vi "Lissage de signal_base_GJE.vi"() -> ()   [LabVIEW 2018]
panel:
  in  "stop":bool
  out "Graphe déroulant":cluster{dbl, dbl, dbl}(graph)
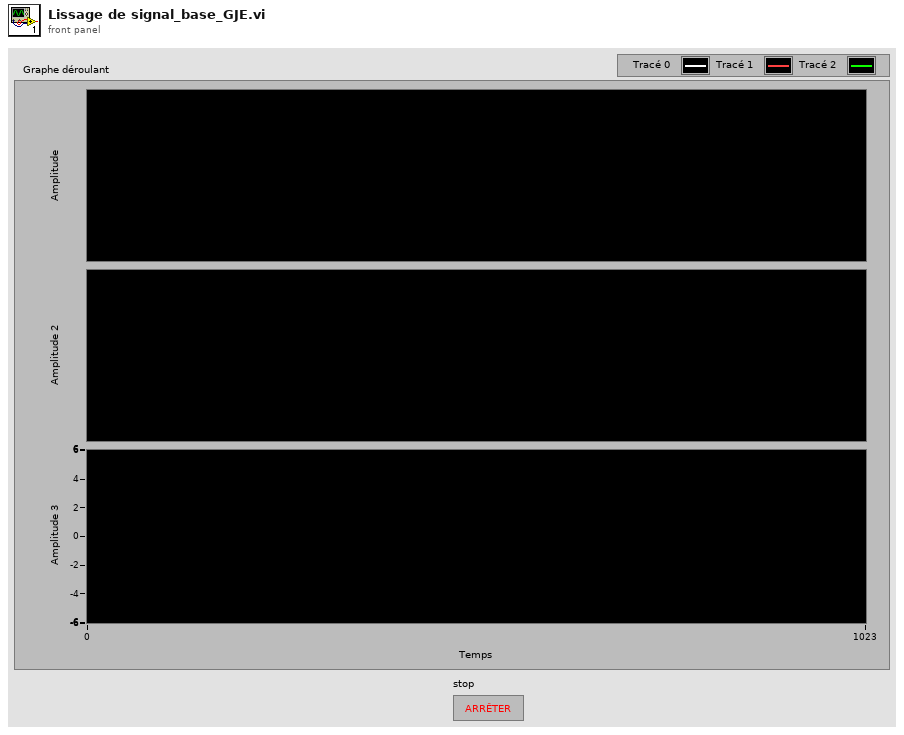
[diagram p1: front panel]
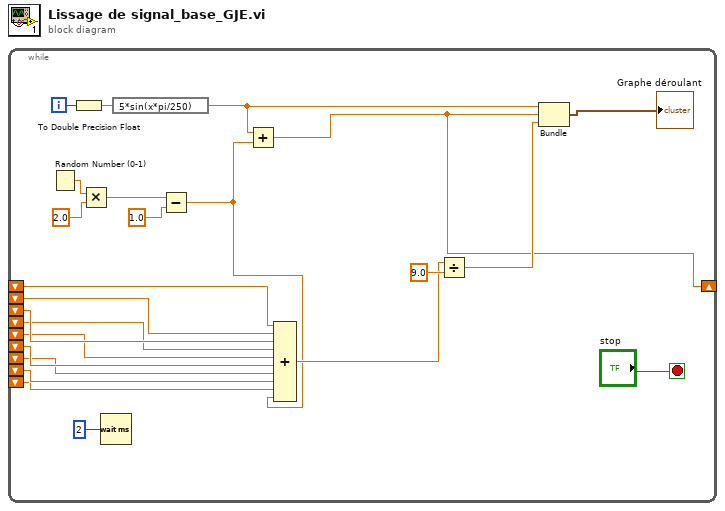
[diagram p0: block diagram]
diagram:
  n1 = while {
    shift-right: [w2] -> _
    shift-left: _ -> [w15]
    shift-left: _ -> [w14]
    shift-left: _ -> [w13]
    shift-left: _ -> [w12]
    shift-left: _ -> [w11]
    shift-left: _ -> [w10]
    shift-left: _ -> [w9]
    shift-left: _ -> [w8]
    shift-left: _ -> [w7]
    i -> [w21]
    stop <- "stop" stop-if-true
    n2 = Random Number (0-1)() -> (number: 0 to 1=w19:dbl)
    n3 = To Double Precision Float(number=w21) -> (double precision float=w23:dbl)
    n4 = Multiply(x=w19, y=2.0) -> (x*y=w17:dbl)
    n5 = Wait (ms)(milliseconds to wait=u32 2 ("attente (ms)")) -> ()  [unwired: 1 out]
    n6 = expression code="5*sin(x*pi/250)"(w23) -> (w16:dbl)
    n7 = Subtract(x=w17, y=1.0) -> (x-y=w1:dbl)
    n8 = Add(x=w16, y=w1) -> (x+y=w2:dbl)
    n9 = Compound Arithmetic op=ADD ("Opérateur arithmétique")(w15, w14, w13, w12, w11, w10, w9, w8, w7, w1) -> (w5:dbl)
    n10 = Divide(x=w5, y=9.0) -> (x/y=w4:dbl)
    n11 = Bundle(w16, w2, w4) -> (→"Graphe déroulant":cluster{dbl, dbl, dbl})  [unwired: 1 in]
  }
